vi "isRefValid.vi"(8 "error in (no error)":errorcluster, 11 "xwpfTable in":refnum<class "xwpfTable.lvclass">) -> (0 "error out":errorcluster, 3 "xwpfTable out":refnum<class "xwpfTable.lvclass">)   [LabVIEW 2017, in "Word_Specific.lvlib" / "xwpfTable.lvclass"]
uses:
  xwpfTable.lvclass
  xwpfTable.lvclass/xwpfTable.ctl
  <vilib>/Utility/error.llb/Error Cluster From Error Code.vi
  <vilib>/ErrorRing/Error Ring.xnode
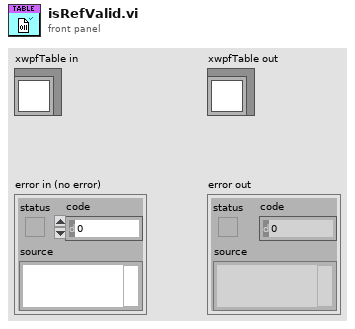
[diagram p1: front panel]
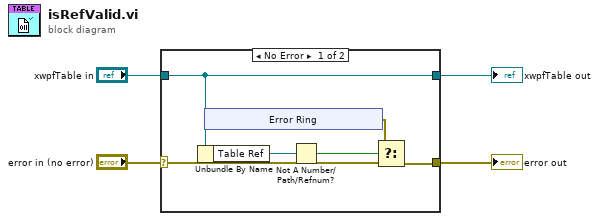
[diagram p0: block diagram]
diagram:
  n1 = case shown="No Error" "error in (no error)" {
    selector: "error in (no error)" -> [w7 w17]
    tunnel: [w6 w17] -> w2
    tunnel: [w10 w16] -> w3
    tunnel: "xwpfTable in" -> [w10 w16]
    frame No Error {
      n2 = Unbundle By Name(w10) -> ("Table Ref"=w5:refnum<k24>)
      n3 = xnode "Error Ring"() -> ("error out"=w8:errorcluster)
      n4 = Not A Number/Path/Refnum?(number/path/refnum=w5) -> (NaN/Path/Refnum?=w9:bool)
      n5 = Select(t=w8, s=w9, f=w7) -> (s? t:f=w6:errorcluster)
    }
    frame Error {
    }
  }
  "error out" <- w2
  "xwpfTable out" <- w3
